vi "Control joystick (SubVI).vi"(2 "Start/stop":bool, 3 "error in (no error)":errorcluster, 5 "VISA Refnum in":refnum<visa-resource-name>) -> (0 "error out":errorcluster, 1 "VISA resource name out":refnum<visa-resource-name>)   [LabVIEW 2018]
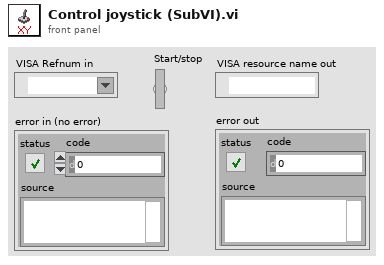
[diagram p1: front panel]
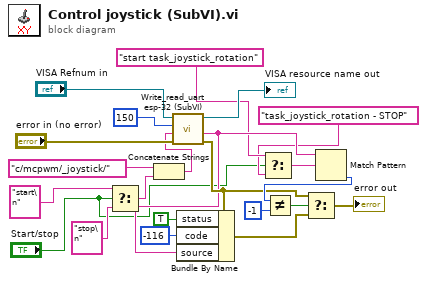
[diagram p0: block diagram]
diagram:
  n1 = Select(t="start\n", s="Start/stop", f="stop\n") -> (s? t:f=w7:string)
  n2 = Concatenate Strings("c/mcpwm/_joystick/" ("write buffer"), w7) -> (w6:string)
  n3 = call "Write_read_uart esp-32 (SubVI).vi"("error in (no error)"="error in (no error)", "write buffer"=w6, "milliseconds to wait"=u32 150, "VISA Refnum in"="VISA Refnum in") -> ("error out 4"=w13:errorcluster, "read buffer"=w5:string, "VISA resource name out"=→"VISA resource name out":refnum<visa-resource-name>)  [unwired: 1 out]
  n4 = Bundle By Name(cluster=w13, "status"=TRUE, "code"=i16 -116, "source"=w5) -> (w12:errorcluster)
  n5 = Select(t="start task_joystick_rotation" ("regular expression"), s="Start/stop", f="task_joystick_rotation - STOP") -> (s? t:f=w4:string)
  n6 = Match Pattern(string=w5, regular expression=w4) -> (offset past match=w17:i32)  [unwired: 1 in, 3 out]
  n7 = Not Equal?(x=w17, y=-1 ("offset past match")) -> (x != y?=w16:bool)
  n8 = Select(t=w13, s=w16, f=w12) -> (s? t:f=→"error out":errorcluster)
